vi "Constants.vi"() -> ()   [LabVIEW 2018, in "Vires VTD Shared.lvlib"]
doc: "Use this Global VI to access the GUIDs assigned to the page resources of the Custom Device."
uses:
  Vires VTD Shared.lvlib
  RDB/RDB Object.ctl
  RDB/RDB Player Object.ctl
  Network Settings.ctl
  Protocol.ctl
  RDB/RDB.lvlib
panel:
  in  "Tab Control":enum32{"GUIDS", "Constants", "Properties"}(tab)=enum."Properties"
  in  "Custom SCP Command Page":string="a74b8f30-7919-4e49-b0a8-0a995d19792c"
  in  "Scenario Selection Page":string="9a66d7b2-5877-47ad-af27-ff67d1338762"
  in  "Generic Channel":string="67e8cc4e-c6f3-4f9e-89c6-959629af069a"
  in  "Simulation Time Page":string="04a2836d-e5e6-4863-a17e-ba936490a375"
  in  "Status Command Page":string="c9af40a3-0f6c-479e-bf1f-8e920242783a"
  in  "Status Error Page":string="e6604a1e-ac70-4f52-887c-1c84b4d0fede"
  in  "Status Time Page":string="7010c573-acbe-46a4-a0eb-2dfca4172be4"
  in  "Status Channel Page":string="1c5c4ba3-58c3-4b06-8594-037c48e58688"
  in  "Vires VTD disabled":string="60592157-0220-4fd1-bb66-4eab64c0d69b"
  in  "Object Page":string="e1239479-4dd4-4df4-8c6a-7421ee36a88f"
  in  "Sensor Page":string="e3955479-4dd4-4df4-8c6a-7421ee36a88f"
  in  "ModuleManager":string="e3955479-4dd4-4df4-8c6a-7421ee36a72e"
  in  "TaskControl":string="e3955479-4dd4-4df4-8c6a-7421ee36a71e"
  in  "Status Page":string="e1234479-4dd4-4df4-ffff-7421ee36a79e"
  in  "Control Page":string="e1234479-4dd4-4df4-8c6a-7421ee36a79e"
  in  "Data Page":string="e3955479-4dd4-4df4-8c6a-7421ee36a79e"
  in  "Structure Section":string="b065f6f6-976e-46c5-4882-eaf4c0fa7449"
  in  "Sent":string="b065f6f6-976e-46c5-ac29-eaf4c0fa7449"
  in  "Receive":string="e1234579-4dd4-4df4-8c6a-7421ee36a79e"
  in  "Vires VTD":string="353f2512-b107-4c99-9510-7a0eded912f5"
  out "Array":T1[](array[typedef])
  in  "RDB Signalname":string
  in  "Default Network Settings":T3={"IP adress"="0.0.0.0", "RDB"={"Protocol"=enum."TCP", "Tx Port"=48191, "Rx Port"=48190, "Buffer Size"=204800, "Timeout"=10}, "SCP"={"Protocol"=enum."TCP", "Tx Port"=48179, "Rx Port"=48179, "Buffer Size"=204800, "Timeout"=60}}
  in  "Custom SCP Formatting":string="Custom SCP Formatting"
  in  "Custom SCP Commands List":string="Custom SCP Commands List"
  in  "Scenario List":string="Scenario List"
  in  "Network Settings":string="Network Settings"
  in  "Network Tab":string="Tab Control"
  # "#todo_ok: not used any more"
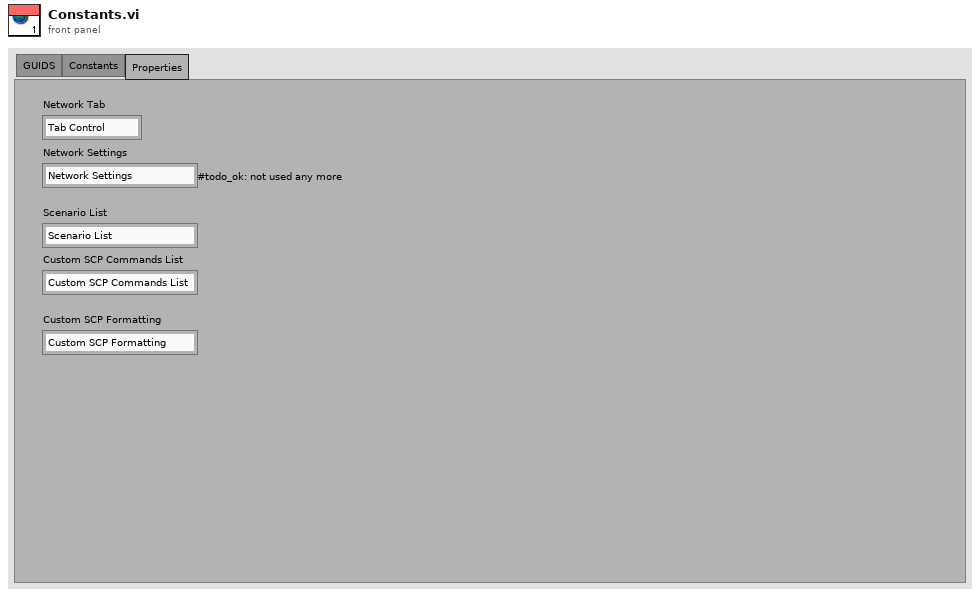
[diagram p1: front panel]
types:
  T1 = typedef "RDB.lvlib/RDB Object.ctl" = cluster{"pkID":i32, "RDB Player Objects":T2[]}
  T2 = typedef "RDB.lvlib/RDB Player Object.ctl" = cluster{"PlayerID":i32, "Signals":string[], "WheelID":i32}
  T3 = typedef "Vires VTD Shared.lvlib/Network Settings.ctl" = cluster{"IP adress":string, "RDB":cluster{"Protocol":T4, "Tx Port":u16, "Rx Port":u16, "Buffer Size":i32, "Timeout":u16}, "SCP":cluster{"Protocol":T4, "Tx Port":u16, "Rx Port":u16, "Buffer Size":i32, "Timeout":u16}}
  T4 = typedef "Vires VTD Shared.lvlib/Protocol.ctl" = enum16{"UDP", "TCP"}
diagram:
